vi "Set Primary Key.vi"(8 "error in (no error)":errorcluster, 10 "Is a PK? (T)":bool=TRUE, 11 "Basic Column Configuration in":refnum<class "Base Column Configuration.lvclass">) -> (0 "error out":errorcluster, 3 "Basic Column Configuration out":refnum<class "Base Column Configuration.lvclass">)   [LabVIEW 2020, in "Column Interfaces.lvlib" / "Base Column Configuration.lvclass"]
uses:
  Base Column Configuration.lvclass
  Base Column Configuration.lvclass/Base Column Configuration.ctl
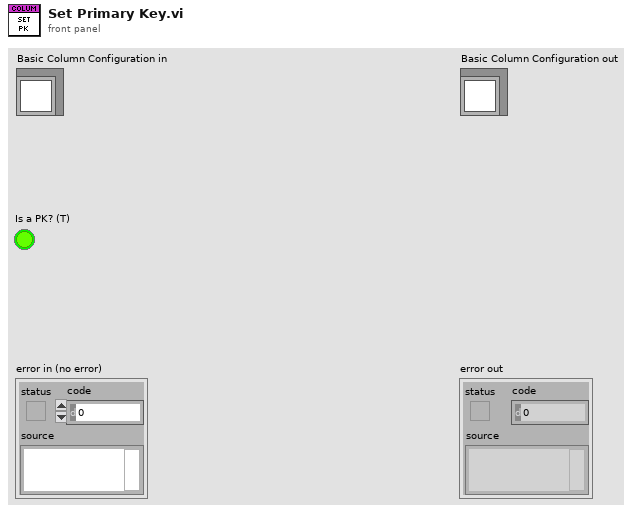
[diagram p1: front panel]
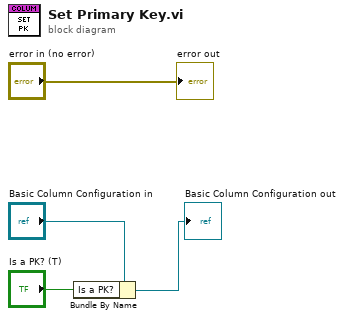
[diagram p0: block diagram]
diagram:
  n1 = Bundle By Name(cluster="Basic Column Configuration in", "Is a PK?"="Is a PK? (T)") -> (→"Basic Column Configuration out":refnum<class "Base Column Configuration.lvclass">)
  "error out" <- "error in (no error)"
